vi "IMAQdx_GetCameraAllAttributes.vi"(8 "error in (no error)":errorcluster caption="错误输入（无错误）", 10 "当前可用相机":string(combo), 11 "表格控件引用_输入":refnum<vi>) -> (0 "error out":errorcluster caption="错误输出", 3 "表格控件引用输出":refnum<vi>)   [LabVIEW 2018]
uses:
  <vilib>/vision/driver/IMAQdx.llb/IMAQdx Attribute Visibility.ctl
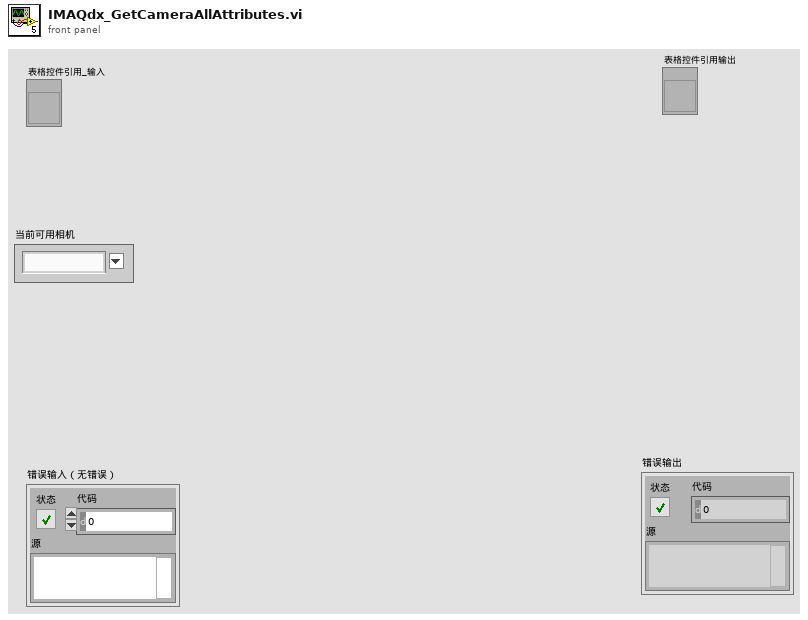
[diagram p1: front panel]
types:
  T1 = typedef "NI_Vision_Acquisition_Software.lvlib/IMAQdx Attribute Visibility.ctl" = enum32{"Simple", "Intermediate", "Advanced"}
  T2 = typedef "IMAQdx.ctl" = refnum<k21>
  T3 = typedef "NI_Vision_Acquisition_Software.lvlib/IMAQdx Attribute Type.ctl" = enum32{"U32", "I64", "DBL", "String", "Enum", "Bool", "Command"}
  T4 = cluster{"Attribute Type":T3, "Readable":bool, "Writable":bool, "Attribute Name":string}[]
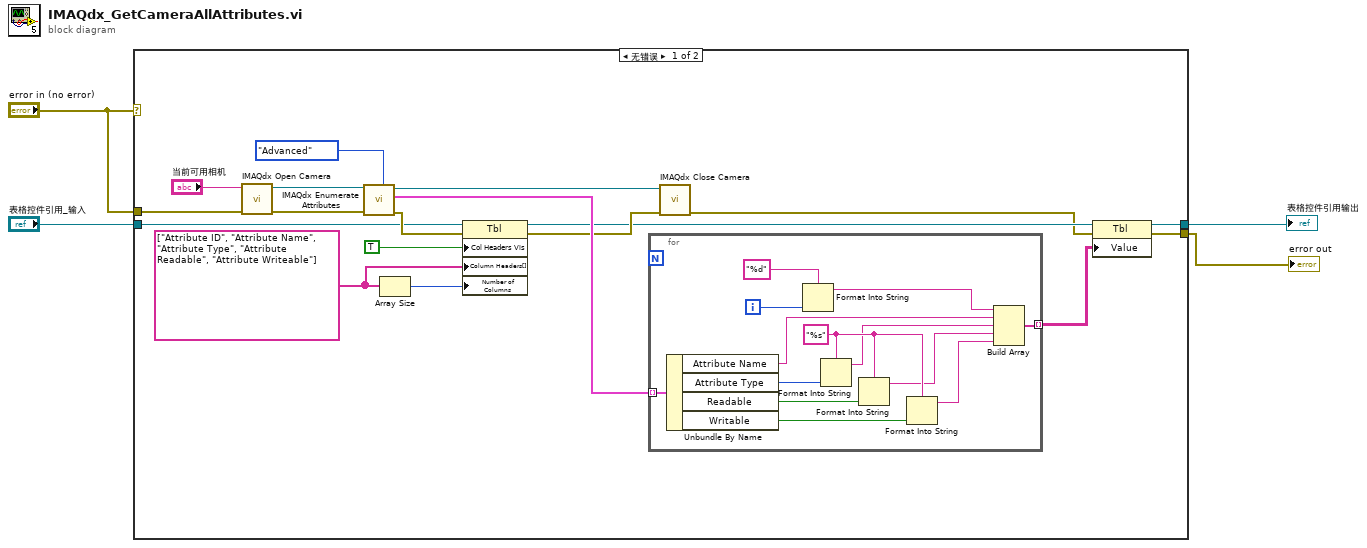
[diagram p0: block diagram]
diagram:
  n1 = case shown="无错误" "error in (no error)" {
    tunnel: "表格控件引用_输入" -> [w14 w37]
    tunnel: [w8 w37] -> w3
    tunnel: "error in (no error)" -> [w9 w36]
    tunnel: [w5 w36] -> w1
    frame No Error {
      w11 = string[] ["Attribute ID", "Attribute Name", "Attribute Type", "Attribute Readable", "Attribute Writeable"]
      n2 = call <vilib>:"IMAQdx Open Camera.vi"("error in"=w9, "Session In"="当前可用相机") -> ("error out"=w21:errorcluster, "Session Out"=w20:T2)  [unwired: 8 in]
      n3 = call <vilib>:"IMAQdx Enumerate Attributes.vi"("Visibility"=IMAQdx_Attribute_Visibility."Advanced", "error in"=w21, "Session In"=w20) -> ("error out"=w16:errorcluster, "Attribute Information Array"=w17:T4, "Session Out"=w19:T2)  [unwired: 6 in]
      n4 = Array Size(array=w11) -> (size(s)=w10:i32)
      n5 = property class="Tbl"(reference=w14, error in=w16, "Col Headers Vis"=TRUE ("显示项:显示列首"), "Column Headers[]"=w11, "Number of Columns"=w10) -> (reference out=w13:refnum<vi>, error out=w15:errorcluster)
      n6 = for {
        tunnel: w17 -> [w35] mode=indexing
        tunnel: [w23] -> w7 mode=indexing
        i -> [w30]
        w31 = "%s" ("格式字符串")
        n7 = Unbundle By Name(w35) -> ("Attribute Name"=w26:string, "Attribute Type"=w34:T3, "Readable"=w33:bool, "Writable"=w32:bool)
        n8 = Format Into String(format string="%d" ("格式字符串"), w30) -> (resulting string=w27:string)  [unwired: 2 in, 1 out]
        n9 = Format Into String(format string=w31, w34) -> (resulting string=w28:string)  [unwired: 2 in, 1 out]
        n10 = Format Into String(format string=w31, w33) -> (resulting string=w25:string)  [unwired: 2 in, 1 out]
        n11 = Format Into String(format string=w31, w32) -> (resulting string=w24:string)  [unwired: 2 in, 1 out]
        n12 = Build Array(w27, w26, w28, w25, w24) -> (w23:string[])
      }
      n13 = call <vilib>:"IMAQdx Close Camera.vi"("error in"=w15, "Session In"=w19) -> ("error out"=w6:errorcluster)  [unwired: 9 in]
      n14 = property class="Tbl"(reference=w13, error in=w6, "Value"=w7) -> (reference out=w8:refnum<vi>, error out=w5:errorcluster)
    }
    frame Error {
    }
  }
  "error out" <- w1
  "表格控件引用输出" <- w3
